vi "Save Current Lighting.vi"(8 "error in (no error)":errorcluster) -> (0 "error out":errorcluster)   [LabVIEW 2022 SP3, in "Logitech Devices.lvlib"]
uses:
  Logitech Devices.lvlib
  <vilib>/Utility/error.llb/Error Cluster From Error Code.vi
  C:/Program Files/LGHUB/sdks/sdk_legacy_led_x86.dll
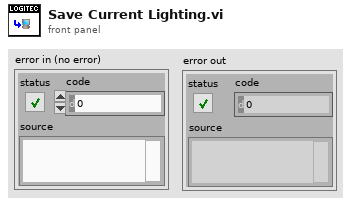
[diagram p1: front panel]
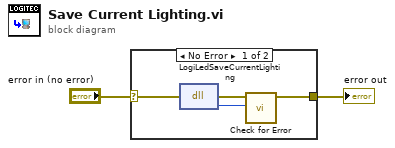
[diagram p0: block diagram]
diagram:
  n1 = case shown="No Error" "error in (no error)" {
    selector: "error in (no error)" -> [w6 w7]
    tunnel: [w3 w7] -> w1
    frame No Error {
      n2 = dll-call lib="C:/Program Files/LGHUB/sdks/sdk_legacy_led_x86.dll" fn="LogiLedSaveCurrentLighting"(error in=w6) -> (error out=w4:errorcluster, "return type"=w5:u8)  [unwired: 2 in, 1 out]
      n3 = call "Check for Error.vi"("DLL-call return value"=w5, "error in (no error)"=w4) -> ("error out"=w3:errorcluster)  [unwired: 9 in]
    }
    frame Error {
    }
  }
  "error out" <- w1
